vi "Untitled 1.vi"() -> ()   [LabVIEW 2021]
uses:
  <instrlib>/Tektronix TDS 200 1000 2000 Series/Public/Configure/Configure Trigger (Edge).vi
  <instrlib>/Tektronix TDS 200 1000 2000 Series/Public/Data/Read (Single Waveform).vi
  <instrlib>/Tektronix TDS 200 1000 2000 Series/Tektronix TDS 200 1000 2000 Series.lvlib
panel:
  in  "Force Manual Trigger":bool
  in  "Acquisition Type (0: Sample)":i32(ring) items=["Sample", "Average", "Peak Detect"]
  in  "error in (no error)":errorcluster
  in  "VISA resource name":refnum<visa-resource-name>
  in  "Trigger Coupling (0: AC)":i32(ring) items=["AC", "DC", "HF Reject", "LF Reject", "Noise Reject"]
  in  "Holdoff (0.00)":dbl format="%_3g"
  in  "Trigger Slope (0: Rising)":i32(ring) items=["Rising", "Falling"]
  in  "Trigger Source (0: Channel 1)":i32(ring) items=["Channel 1", "Channel 2", "Channel 3", "Channel 4", "External Input", "Attenuated External Input"]
  in  "Trigger Level (0.0 V)":dbl
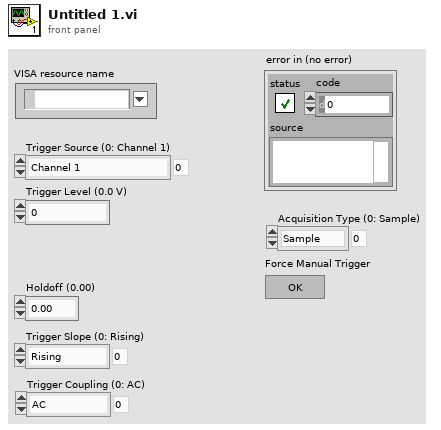
[diagram p1: front panel]
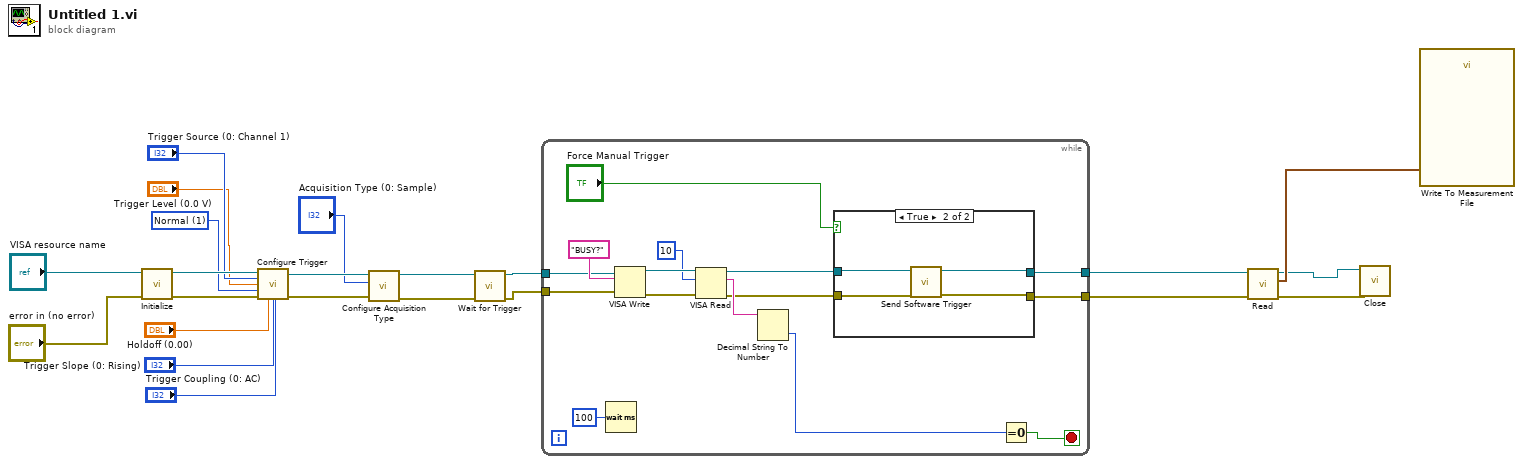
[diagram p0: block diagram]
diagram:
  w5 = 1 items=["Auto", "Normal"] ("Trigger Mode (0: Auto)")
  n1 = call <instrlib>:"Initialize.vi"("error in (no error)"="error in (no error)", "VISA resource name"="VISA resource name") -> ("error out"=w19:errorcluster, "VISA resource name out"=w20:refnum<visa-resource-name>)  [unwired: 8 in]
  n2 = call-poly <instrlib>:"Configure Trigger.vi"("VISA resource name"=w20, "Trigger Source (0: Channel 1)"="Trigger Source (0: Channel 1)", "Trigger Level (0.0 V)"="Trigger Level (0.0 V)", "Trigger Mode (0: Auto)"=w5, "error in (no error)"=w19, "Holdoff (0.00)"="Holdoff (0.00)", "Trigger Slope (0: Rising)"="Trigger Slope (0: Rising)", "Trigger Coupling (0: AC)"="Trigger Coupling (0: AC)") -> ("VISA resource name out"=w22:refnum<visa-resource-name>, "error out"=w21:errorcluster)  [unwired: 6 in]
  n3 = call <instrlib>:"Configure Acquisition Type.vi"("error in (no error)"=w21, "Acquisition Type (0: Sample)"="Acquisition Type (0: Sample)", "VISA resource name"=w22) -> ("error out"=w9:errorcluster, "VISA resource name out"=w10:refnum<visa-resource-name>)  [unwired: 7 in]
  n4 = call <instrlib>:"Wait for Trigger.vi"("error in (no error)"=w9, "VISA resource name"=w10) -> ("error out"=w3:errorcluster, "VISA resource name out"=w4:refnum<visa-resource-name>)  [unwired: 8 in]
  n5 = while {
    tunnel: w4 -> [w29]
    tunnel: w3 -> [w28]
    tunnel: [w24] -> w2
    tunnel: [w23] -> w1
    stop <- w30 stop-if-true
    n6 = Wait (ms)(milliseconds to wait=u32 100) -> ()  [unwired: 1 out]
    n7 = VISA Write(VISA resource name=w29, write buffer="BUSY?", error in (no error)=w28) -> (VISA resource name out=w34:refnum<visa-resource-name>, error out=w35:errorcluster)  [unwired: 1 out]
    n8 = VISA Read(VISA resource name=w34, byte count=u32 10, error in (no error)=w35) -> (VISA resource name out=w26:refnum<visa-resource-name>, read buffer=w36:string, error out=w25:errorcluster)  [unwired: 1 out]
    n9 = Decimal String To Number(string=w36) -> (number=w31:i32)  [unwired: 2 in, 1 out]
    n10 = case shown="True" "Force Manual Trigger" {
      tunnel: w26 -> [w39 w43]
      tunnel: w25 -> [w38 w42]
      tunnel: [w39 w41] -> w24
      tunnel: [w38 w40] -> w23
      frame False {
      }
      frame True {
        n11 = call <instrlib>:"Send Software Trigger.vi"("error in (no error)"=w42, "VISA resource name"=w43) -> ("error out"=w40:errorcluster, "VISA resource name out"=w41:refnum<visa-resource-name>)  [unwired: 8 in]
      }
    }
    n12 = Equal To 0?(x=w31) -> (x = 0?=w30:bool)
  }
  n13 = call-poly <instrlib>:"Read.vi"("error in (no error)"=w1, "VISA resource name"=w2) -> ("error out"=w6:errorcluster, "Waveform Data"=w8:waveform(dbl), "VISA resource name out"=w7:refnum<visa-resource-name>)  [unwired: 7 in]
  n14 = call <instrlib>:"Close.vi"("error in (no error)"=w6, "VISA resource name"=w7) -> ()  [unwired: 9 in, 1 out]
  n15 = call "Write To Measurement File"("Signals"=w8) -> ()  [unwired: 16 in, 3 out]
